vi "update_component.vi"(8 "error in (no error)":errorcluster, 10 "Component":T1, 11 "DB Session ID":i32) -> (0 "error out":errorcluster, 2 "Component out":T1, 3 "DB Session ID out":i32)   [LabVIEW 2023, in "Database.lvlib"]
uses:
  Database.lvlib
  DB Component.ctl
  bin/Database.dll
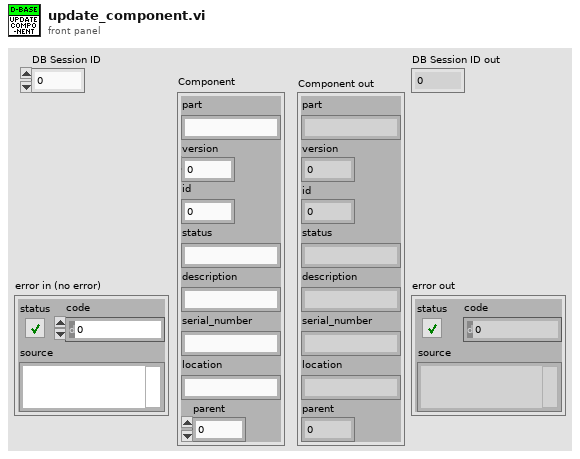
[diagram p1: front panel]
types:
  T1 = typedef "Database.lvlib/DB Component.ctl" = cluster{"part":string, "version":i32, "id":i32, "status":string, "description":string, "serial_number":string, "location":string, "parent":i32}
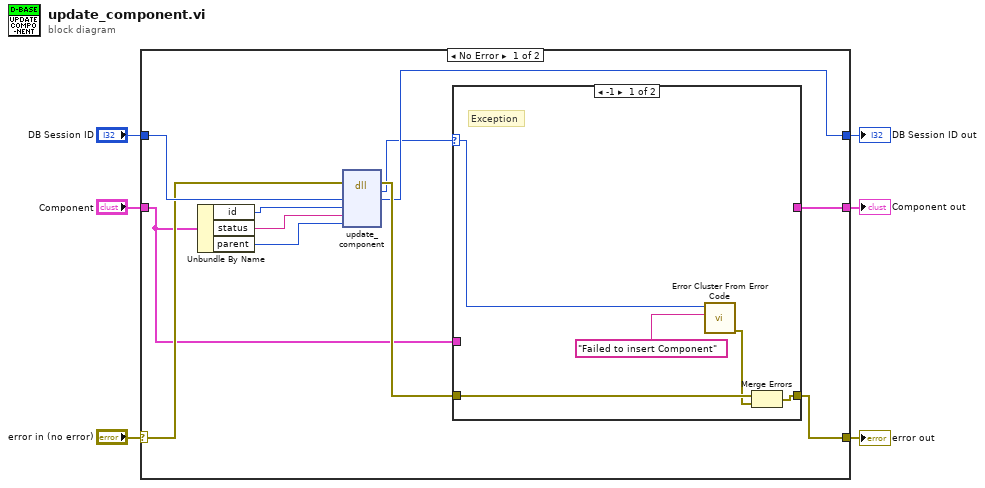
[diagram p0: block diagram]
diagram:
  n1 = case shown="No Error" "error in (no error)" {
    selector: "error in (no error)" -> [w15 w27]
    tunnel: [w14 w27] -> w4
    tunnel: "DB Session ID" -> [w16 w26]
    tunnel: [w13 w25] -> w1
    tunnel: [w12 w26] -> w3
    tunnel: "Component" -> [w11 w25]
    frame No Error {
      n2 = Unbundle By Name(w11) -> ("id"=w9:i32, "status"=w10:string, "parent"=w8:i32)
      n3 = dll-call lib="C:/Users/cfangmeier3/Desktop/nebraska-silicon-lab/pixel-gantry-control/Gantry/Shared Components/bin/Database.dll" fn="update_component"(error in=w15, "conn_id"=w16, "id"=w9, "status"=w10, "parent"=w8) -> (error out=w17:errorcluster, "return type"=w7:i32, "conn_id"=w12:i32)  [unwired: 5 in, 1 out]
      n4 = case shown="-1" w7 {
        selector: w7 -> [w18 _]
        tunnel: w17 -> [w22 w24]
        tunnel: [w21 w24] -> w14
        tunnel: [_ w23] -> w13
        tunnel: w11 -> [_ w23]
        frame -1 {
          # "Exception"
          n5 = call <vilib>:"Error Cluster From Error Code.vi"("error message (\"\")"="Failed to insert Component" ("error message (\"\")"), "error code (0)"=w18) -> ("error out"=w20:errorcluster)  [unwired: 7 in]
          n6 = Merge Errors(w22, w20) -> (w21:errorcluster)
        }
        frame Default {
          # "Ok"
        }
      }
    }
    frame Error {
    }
  }
  "error out" <- w4
  "DB Session ID out" <- w3
  "Component out" <- w1
